vi "Computer.vi"() -> ()   [LabVIEW 2013]
uses:
  <vilib>/Utility/inputDevices.llb/closeJoystick.vi
  <vilib>/Utility/inputDevices.llb/joystickAcquire.vi
panel:
  in  "Robot Port":u16=2055 min=1025 step=1
  in  "Robot Address":string="192.168.1.200"
  in  "stop":bool
  in  "ESTOP":bool
  out "TX Data":T1
  # "Computer Control"
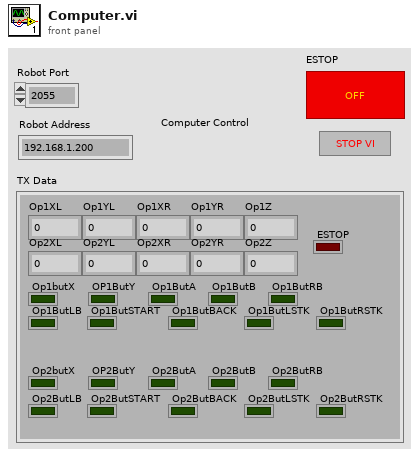
[diagram p1: front panel]
types:
  T1 = cluster{"Op2ButLSTK":bool, "Op2ButRSTK":bool, "Op1ButLSTK":bool, "Op1ButRSTK":bool, "Op1XL":i32, "Op1YL":i32, "Op1XR":i32, "Op1YR":i32, "Op1Z":i32, "Op2XL":i32, "Op2YL":i32, "Op2XR":i32, "Op2YR":i32, "Op2Z":i32, "ESTOP":bool, "Op1butX":bool, "OP1ButY":bool, "Op1ButA":bool, "Op1ButB":bool, "Op1ButRB":bool, "Op1ButLB":bool, "Op2butX":bool, "OP2ButY":bool, "Op2ButA":bool, "Op2ButB":bool, "Op2ButRB":bool, "Op2ButLB":bool, "Op2ButSTART":bool, "Op2ButBACK":bool, "Op1ButSTART":bool, "Op1ButBACK":bool}
  T2 = cluster{"X axis":i32, "Y axis":i32, "Z axis":i32, "X axis rotation":i32, "Y axis rotation":i32, "Z axis rotation":i32, "U axis":i32, "V axis":i32}
  T3 = cluster{"button 1":bool, "button 2":bool, "button 3":bool, "button 4":bool, "button 5":bool, "button 6":bool, "button 7":bool, "button 8":bool, "button 9":bool, "button 10":bool, "button 11":bool, "button 12":bool, "button 13":bool, "button 14":bool, "button 15":bool, "button 16":bool, "button 17":bool, "button 18":bool, "button 19":bool, "button 20":bool, "button 21":bool, "button 22":bool, "button 23":bool, "button 24":bool, "button 25":bool, "button 26":bool, "button 27":bool, "button 28":bool, "button 29":bool, "button 30":bool, "button 31":bool, "button 32":bool}
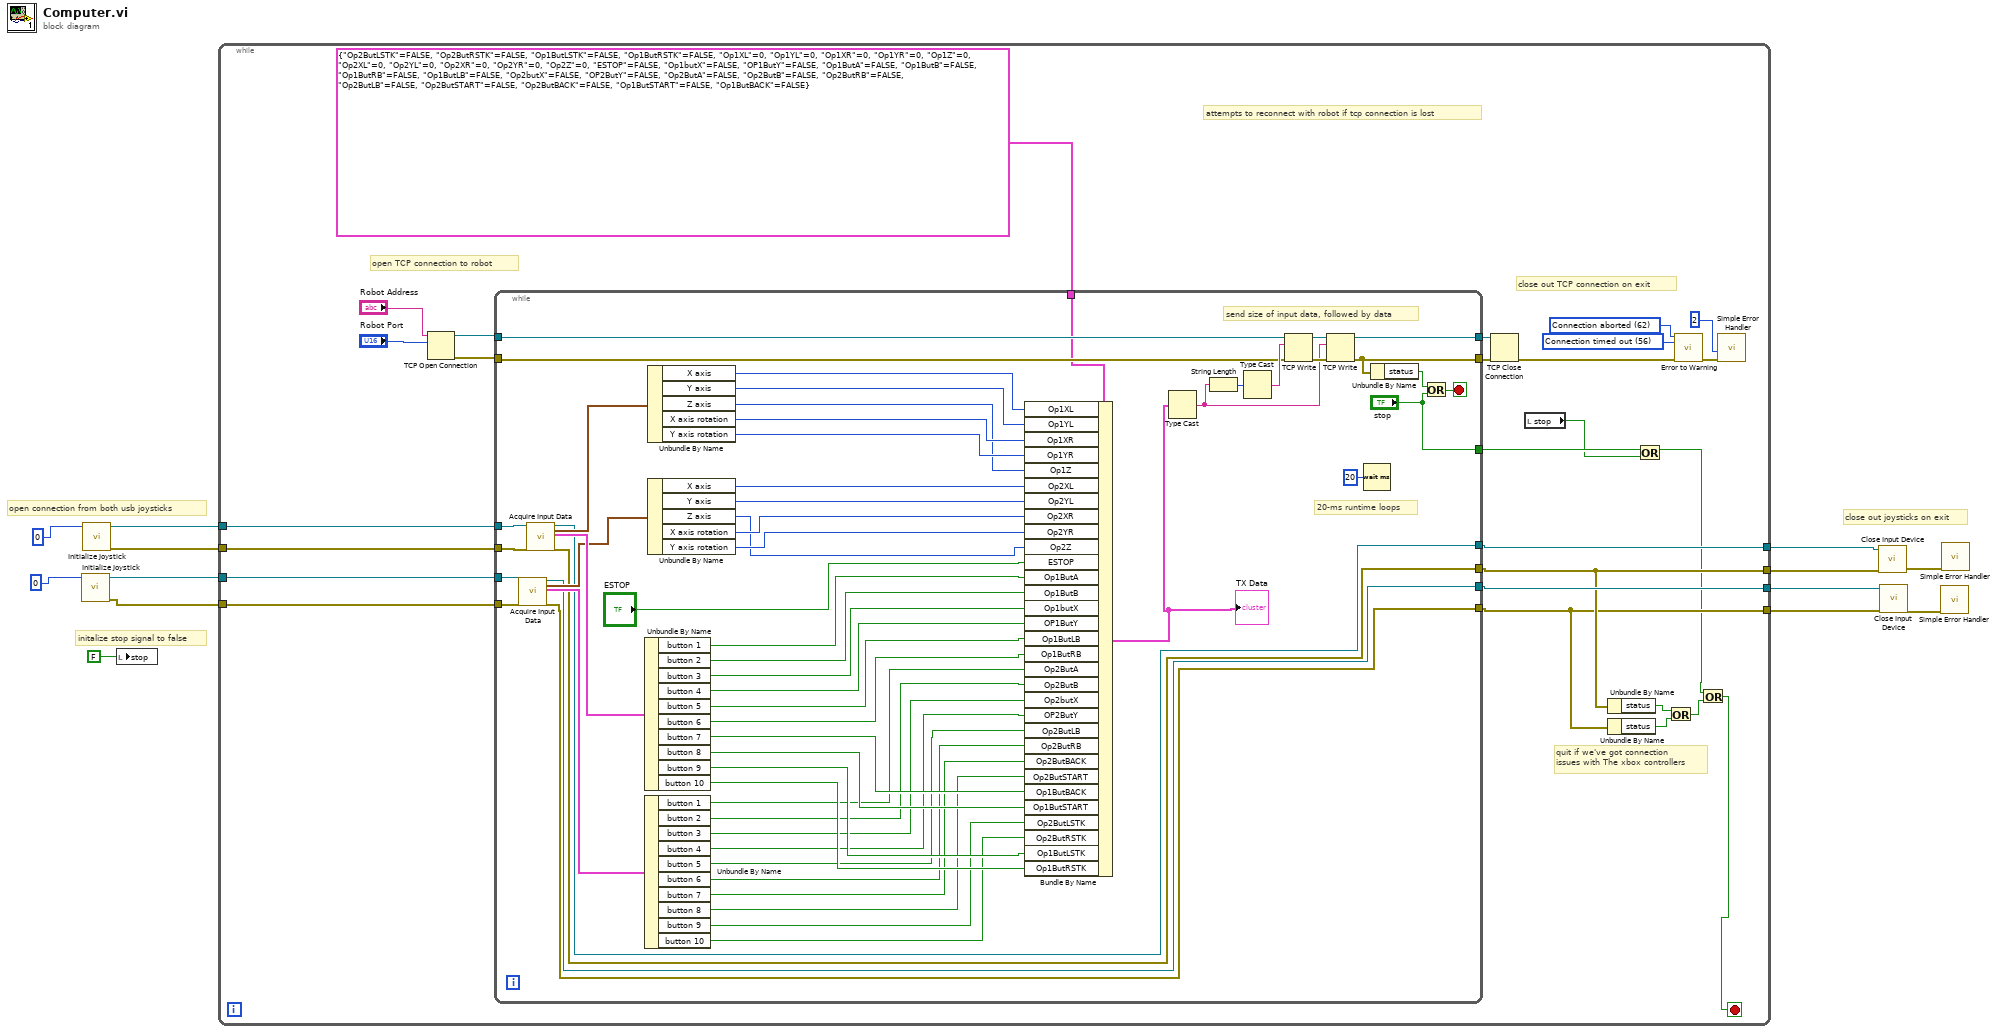
[diagram p0: block diagram]
diagram:
  # "initalize stop signal to false"
  # "open connection from both usb joysticks"
  # "close out joysticks on exit"
  n1 = call <vilib>:"Initialize Joystick.vi"("device index"=0) -> ("error out"=w2:errorcluster, "device ID"=w3:refnum<k1>)  [unwired: 9 in]
  n2 = call <vilib>:"Initialize Joystick.vi"("device index"=0) -> ("error out"=w4:errorcluster, "device ID"=w5:refnum<k1>)  [unwired: 9 in]
  n3 = local write "stop"(FALSE) -> ()
  n4 = while {
    tunnel: [w29] -> w11
    tunnel: [w27] -> w10
    tunnel: [w28] -> w9
    tunnel: [w26] -> w8
    tunnel: w5 -> [w20]
    tunnel: w4 -> [w19]
    tunnel: w3 -> [w18]
    tunnel: w2 -> [w17]
    stop <- w21 stop-if-true
    w37 = 56 items=["No Error", "Argument Error", "Memory Full", "Out of Zone", "End of File", "File Already Open", "Generic File IO Error", "File Not Found", "File Permission Error", "Disk Full", "Duplicate Path", "Too Many Files Open", "Not Enabled", "Resource File Not Found", "Cannot Add Resource", "Resource Not Found", "Image Not Found", "Image Memory Error", "Pen Does Not Exist", "Config Bad Type", "Config Token Not Found", "Config Parse Error", "Config Memory Error", "Bad External Code Format", "Bad External Code Offset", "External Code Not Present", "Null Window", "Destroy Window Mixup", "Null Menu", "Print Aborted", "Bad Print Record", "Print Driver Error", "Windows Error During Print", "Memory Error During Print", "Print Dialog Error", "Generic Print Error", "Invalid Device Refnum", "Device Not Found", "Device Parameter Error", "Device Unit Error", "Can't Open Device", "Device Call Aborted", "Generic Error", "Cancelled By User", "Object ID Too Low", "Object ID Too High", "Object Not In Heap", "Unknown Heap", "Bad DefProc ID", "DefProc Not In Table", "Message Out Of Range", "Null Method", "Unknown Message", "Manager Call Not Supported", "Bad address", "Connection In progress", "Connection timed out", "Connection is already in progress", "Network attribute not supported", "Network error", "Address in use", "System out of memory", "Connection aborted", "Connection refused", "Connection is not connected", "Connection is already connected", "Connection closed", "Initialize error (interapplication manager)", "Bad occurrence", "Wait on unbound occurrence handler", "Occurrence queue overflow", "Bad path", "Semaphore not signaled", "Unrecognized type (interapplication manager)"] ("2nd Error to Convert")
    w38 = 62 items=["No Error", "Argument Error", "Memory Full", "Out of Zone", "End of File", "File Already Open", "Generic File IO Error", "File Not Found", "File Permission Error", "Disk Full", "Duplicate Path", "Too Many Files Open", "Not Enabled", "Resource File Not Found", "Cannot Add Resource", "Resource Not Found", "Image Not Found", "Image Memory Error", "Pen Does Not Exist", "Config Bad Type", "Config Token Not Found", "Config Parse Error", "Config Memory Error", "Bad External Code Format", "Bad External Code Offset", "External Code Not Present", "Null Window", "Destroy Window Mixup", "Null Menu", "Print Aborted", "Bad Print Record", "Print Driver Error", "Windows Error During Print", "Memory Error During Print", "Print Dialog Error", "Generic Print Error", "Invalid Device Refnum", "Device Not Found", "Device Parameter Error", "Device Unit Error", "Can't Open Device", "Device Call Aborted", "Generic Error", "Cancelled By User", "Object ID Too Low", "Object ID Too High", "Object Not In Heap", "Unknown Heap", "Bad DefProc ID", "DefProc Not In Table", "Message Out Of Range", "Null Method", "Unknown Message", "Manager Call Not Supported", "Bad address", "Connection In progress", "Connection timed out", "Connection is already in progress", "Network attribute not supported", "Network error", "Address in use", "System out of memory", "Connection aborted", "Connection refused", "Connection is not connected", "Connection is already connected", "Connection closed", "Initialize error (interapplication manager)", "Bad occurrence", "Wait on unbound occurrence handler", "Occurrence queue overflow", "Bad path", "Semaphore not signaled", "Unrecognized type (interapplication manager)"] ("1st Error to Convert")
    # "attempts to reconnect with robot if tcp connection is lost"
    # "quit if we've got connection \nissues with The xbox controllers"
    # "close out TCP connection on exit"
    # "open TCP connection to robot"
    n5 = TCP Open Connection(address="Robot Address", remote port or service name="Robot Port") -> (connection ID=w32:refnum<k5>, error out=w31:errorcluster)  [unwired: 3 in]
    n6 = while {
      tunnel: [w90] -> w35
      tunnel: [w98] -> w36
      tunnel: w32 -> [w97]
      tunnel: w31 -> [w87]
      tunnel: w20 -> [w86]
      tunnel: w19 -> [w85]
      tunnel: T1 {"Op2ButLSTK"=FALSE, "Op2ButRSTK"=FALSE, "Op1ButLSTK"=FALSE, "Op1ButRSTK"=FALSE, "Op1XL"=0, "Op1YL"=0, "Op1XR"=0, "Op1YR"=0, "Op1Z"=0, "Op2XL"=0, "Op2YL"=0, "Op2XR"=0, "Op2YR"=0, "Op2Z"=0, "ESTOP"=FALSE, "Op1butX"=FALSE, "OP1ButY"=FALSE, "Op1ButA"=FALSE, "Op1ButB"=FALSE, "Op1ButRB"=FALSE, "Op1ButLB"=FALSE, "Op2butX"=FALSE, "OP2ButY"=FALSE, "Op2ButA"=FALSE, "Op2ButB"=FALSE, "Op2ButRB"=FALSE, "Op2ButLB"=FALSE, "Op2ButSTART"=FALSE, "Op2ButBACK"=FALSE, "Op1ButSTART"=FALSE, "Op1ButBACK"=FALSE} -> [w84]
      tunnel: w18 -> [w47]
      tunnel: w17 -> [w46]
      tunnel: [w45] -> w29
      tunnel: [w44] -> w28
      tunnel: [w43] -> w27
      tunnel: [w42] -> w26
      tunnel: ["stop"] -> w23
      stop <- w89 stop-if-true
      # "send size of input data, followed by data"
      # "20-ms runtime loops"
      n7 = call-poly <vilib>:"Acquire Input Data.vi"("device ID"=w47, "error in (no error)"=w46) -> ("device ID"=w44:refnum<k1>, "axis info"=w48:T2, "button info"=w49:T3, "error out"=w42:errorcluster)  [unwired: 13 in, 1 out]
      n8 = call-poly <vilib>:"Acquire Input Data.vi"("device ID"=w86, "error in (no error)"=w85) -> ("device ID"=w45:refnum<k1>, "axis info"=w67:T2, "button info"=w66:T3, "error out"=w43:errorcluster)  [unwired: 13 in, 1 out]
      n9 = Unbundle By Name(w66) -> ("button 1"=w77:bool, "button 2"=w76:bool, "button 3"=w75:bool, "button 4"=w74:bool, "button 5"=w73:bool, "button 6"=w72:bool, "button 7"=w71:bool, "button 8"=w70:bool, "button 9"=w69:bool, "button 10"=w68:bool)
      n10 = Unbundle By Name(w49) -> ("button 1"=w61:bool, "button 2"=w60:bool, "button 3"=w59:bool, "button 4"=w58:bool, "button 5"=w57:bool, "button 6"=w56:bool, "button 7"=w55:bool, "button 8"=w54:bool, "button 9"=w53:bool, "button 10"=w52:bool)
      n11 = Unbundle By Name(w67) -> ("X axis"=w81:i32, "Y axis"=w80:i32, "Z axis"=w51:i32, "X axis rotation"=w79:i32, "Y axis rotation"=w78:i32)
      n12 = Unbundle By Name(w48) -> ("X axis"=w65:i32, "Y axis"=w64:i32, "Z axis"=w50:i32, "X axis rotation"=w63:i32, "Y axis rotation"=w62:i32)
      n13 = Bundle By Name(cluster=w84, "Op1XL"=w81, "Op1YL"=w80, "Op1XR"=w79, "Op1YR"=w78, "Op1Z"=w51, "Op2XL"=w65, "Op2YL"=w64, "Op2XR"=w63, "Op2YR"=w62, "Op2Z"=w50, "ESTOP"="ESTOP", "Op1ButA"=w77, "Op1ButB"=w76, "Op1butX"=w75, "OP1ButY"=w74, "Op1ButLB"=w73, "Op1ButRB"=w72, "Op2ButA"=w61, "Op2ButB"=w60, "Op2butX"=w59, "OP2ButY"=w58, "Op2ButLB"=w57, "Op2ButRB"=w56, "Op2ButBACK"=w55, "Op2ButSTART"=w54, "Op1ButBACK"=w71, "Op1ButSTART"=w70, "Op2ButLSTK"=w53, "Op2ButRSTK"=w52, "Op1ButLSTK"=w69, "Op1ButRSTK"=w68) -> (w83:T1)
      "TX Data" <- w83
      n14 = Type Cast(x=w83) -> (*(type *) &x=w92:string)  [unwired: 1 in]
      n15 = String Length(string=w92) -> (length=w94:i32)
      n16 = Type Cast(x=w94) -> (*(type *) &x=w93:string)  [unwired: 1 in]
      n17 = TCP Write(connection ID=w97, data in=w93, error in (no error)=w87) -> (connection ID out=w96:refnum<k5>, error out=w95:errorcluster)  [unwired: 1 in, 1 out]
      n18 = TCP Write(connection ID=w96, data in=w92, error in (no error)=w95) -> (connection ID out=w98:refnum<k5>, error out=w90:errorcluster)  [unwired: 1 in, 1 out]
      n19 = Wait (ms)(milliseconds to wait=u32 20) -> ()  [unwired: 1 out]
      n20 = Unbundle By Name(w90) -> ("status"=w88:bool)
      n21 = Or(x=w88, y="stop") -> (x .or. y?=w89:bool)
    }
    n22 = TCP Close Connection(connection ID=w36, error in (no error)=w35) -> (error out=w40:errorcluster)  [unwired: 1 in, 1 out]
    n23 = local read "stop"() -> (w15:bool)
    n24 = Unbundle By Name(w27) -> ("status"=w25:bool)
    n25 = Unbundle By Name(w26) -> ("status"=w24:bool)
    n26 = Or(x=w23, y=w15) -> (x .or. y?=w16:bool)
    n27 = Or(x=w25, y=w24) -> (x .or. y?=w22:bool)
    n28 = call <vilib>:"Error to Warning.vi"("1st Error to Convert"=w38, "2nd Error to Convert"=w37, "error in"=w40) -> ("warning out"=w39:errorcluster)  [unwired: 12 in]
    n29 = Or(x=w16, y=w22) -> (x .or. y?=w21:bool)
    n30 = call <vilib>:"Simple Error Handler.vi"("type of dialog (OK msg:1)"=u32 2 ("milliseconds to wait"), "error in (no error)"=w39) -> ()  [unwired: 3 in, 5 out]
  }
  n31 = call-poly <vilib>:"Close Input Device.vi"("error in (no error)"=w10, "device ID"=w11) -> ("error out"=w12:errorcluster)  [unwired: 8 in]
  n32 = call-poly <vilib>:"Close Input Device.vi"("error in (no error)"=w8, "device ID"=w9) -> ("error out"=w13:errorcluster)  [unwired: 8 in]
  n33 = call <vilib>:"Simple Error Handler.vi"("error in (no error)"=w13) -> ()  [unwired: 4 in, 5 out]
  n34 = call <vilib>:"Simple Error Handler.vi"("error in (no error)"=w12) -> ()  [unwired: 4 in, 5 out]
